vi "A-line sum.vi"(8 "Error in":errorcluster, 11 "data in":sgl[][](array[numeric])=[[1.0, 5.0, 8.0, 4.0, 4.0], [1.0, 5.0, 7.0, 4.0, 3.0], [1.0, 6.0, 8.0, 4.0, 4.0], [1.0, 5.0, 9.0, 4.0, 4.0], [1.0, 6.0, 7.0, 5.0, 3.0]]) -> (0 "Error Out":errorcluster, 1 "Z stage move down(um)":dbl, 2 "surface depth":i32, 3 "focus depth":i32)   [LabVIEW 2018]
panel:
  in  "focus depth":dbl=10.0
  out "gradiant":dbl[](array[numeric])
  out "A-line sum":sgl[](array[numeric])
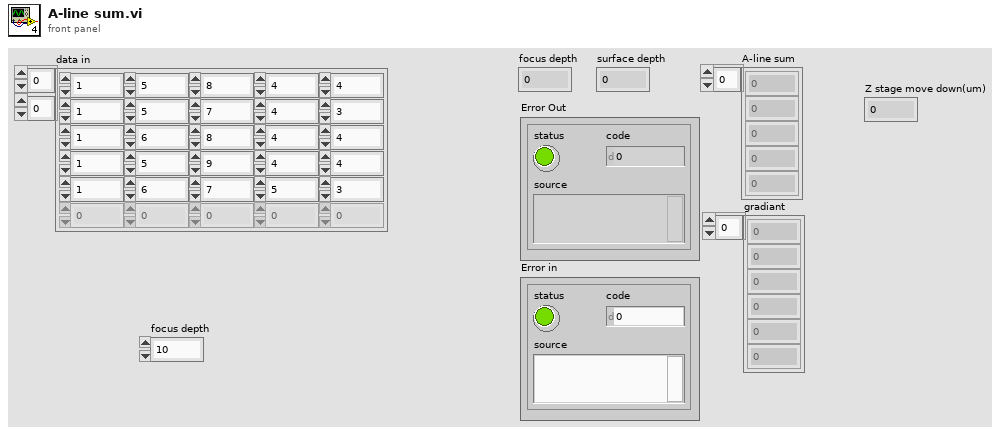
[diagram p1: front panel]
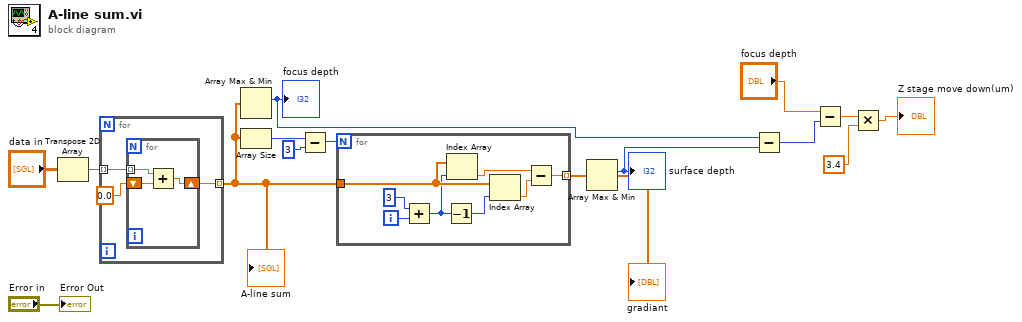
[diagram p0: block diagram]
diagram:
  n1 = Transpose 2D Array(2D array="data in") -> (transposed array=w14:sgl[][])
  n2 = for {
    tunnel: w14 -> [w18] mode=indexing
    tunnel: [w17] -> w12 mode=indexing
    n3 = for {
      tunnel: w18 -> [w21] mode=indexing
      shift-right: [w20] -> w17
      shift-left: 0.0 -> [w19]
      n4 = Add(x=w21, y=w19) -> (x+y=w20:dbl)
    }
  }
  "A-line sum" <- w12
  n5 = Array Max & Min(array=w12) -> (max index (indices)=w7:i32)  [unwired: 3 out]
  "focus depth" <- w7
  n6 = Array Size(array=w12) -> (size(s)=w11:i32)
  n7 = Subtract(x=w11, y=3) -> (x-y=w9:i32)
  n8 = for {
    N: w9 -> [_]
    tunnel: w12 -> [w26]
    tunnel: [w22] -> w8 mode=indexing
    i -> [w29]
    n9 = Add(x=3, y=w29) -> (x+y=w25:i32)
    n10 = Decrement(x=w25) -> (x-1=w27:i32)
    n11 = Index Array(array=w26, index=w25) -> (element=w24:dbl)
    n12 = Index Array(array=w26, index=w27) -> (element=w23:dbl)
    n13 = Subtract(x=w24, y=w23) -> (x-y=w22:dbl)
  }
  "gradiant" <- w8
  n14 = Array Max & Min(array=w8) -> (max index (indices)=w6:i32)  [unwired: 3 out]
  "surface depth" <- w6
  n15 = Subtract(x=w7, y=w6) -> (x-y=w4:i32)
  n16 = Subtract(x="focus depth", y=w4) -> (x-y=w3:dbl)
  n17 = Multiply(x=w3, y=3.4) -> (x*y=→"Z stage move down(um)":dbl)
  "Error Out" <- "Error in"
